vi "project_file_write.vi"(8 "error in (no error)":errorcluster, 10 "project_file":path, 11 "lv-build in":refnum<class "lv-builder-l3.lvclass">) -> (0 "error out":errorcluster, 3 "lv-build out":refnum<class "lv-builder-l3.lvclass">)   [LabVIEW 2015, in "lv-builder-l3.lvlib" / "lv-builder-l3.lvclass"]
uses:
  lv-builder-l3.lvclass
  lv-builder-l3.lvclass/lv-builder-l3.ctl
  lv-builder-l3.lvlib
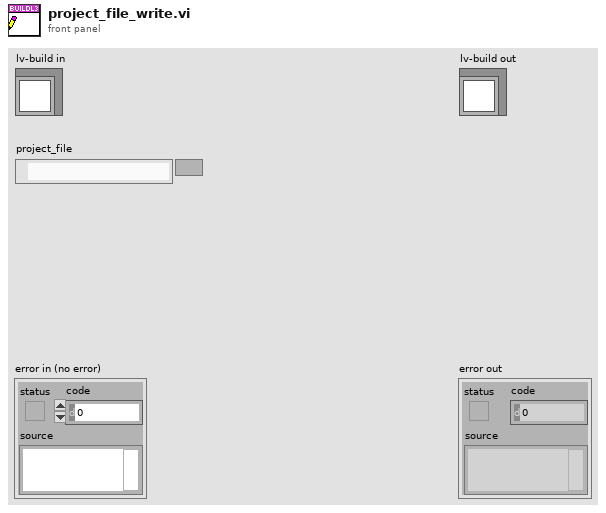
[diagram p1: front panel]
types:
  T1 = typedef "lv-builder-l3.lvlib/configuration.ctl" = cluster{"l3_archive_file_path":string}
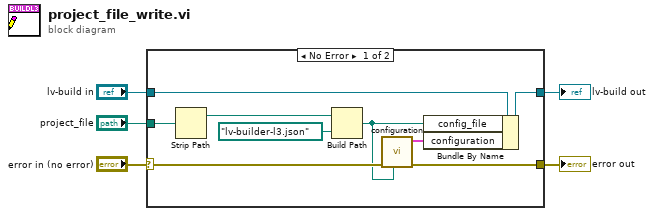
[diagram p0: block diagram]
diagram:
  n1 = case shown="No Error" "error in (no error)" {
    selector: "error in (no error)" -> [w14 w15]
    tunnel: [w6 w15] -> w2
    tunnel: [w9 w16] -> w1
    tunnel: "lv-build in" -> [w13 w16]
    tunnel: "project_file" -> [w10 _]
    frame No Error {
      n2 = Strip Path(path=w10) -> (stripped path=w12:path)  [unwired: 1 out]
      n3 = Build Path(base path=w12, name or relative path=path "lv-builder-l3.json" ("stripped path")) -> (appended path=w7:path)
      n4 = call "configuration.vi"("config_file"=w7, "error in (no error)"=w14) -> ("error out"=w6:errorcluster, "config out"=w8:T1)  [unwired: 8 in]
      n5 = Bundle By Name(cluster=w13, "config_file"=w7, "configuration"=w8) -> (w9:refnum<class "lv-builder-l3.lvclass">)
    }
    frame Error {
    }
  }
  "error out" <- w2
  "lv-build out" <- w1
